vi "2d3dmain.vi"(8 "error in":errorcluster) -> (0 "error out":errorcluster)   [LabVIEW 2023]
uses:
  control/Data Form.ctl
  <vilib>/Utility/miscctls.llb/LVStringsAndValuesArrayTypeDef_U16.ctl
  control/param_calibrazione.ctl
  <vilib>/Analysis/1siggen.llb/Ramp Pattern by Samples.vi
  <vilib>/Utility/file.llb/Read Delimited Spreadsheet (string).vi
  <vilib>/Utility/file.llb/Read Delimited Spreadsheet (DBL).vi
  <vilib>/Utility/file.llb/Write Delimited Spreadsheet (I64).vi
  queue/Front Panel Message Queue.lvlib
  <vilib>/Analysis/NI_AALBase.lvlib
panel:
  in  "Crop Z sl":cluster{i32, i32}(slide) scale=0.0..10.0
  in  "crop Z":bool
  in  "export":bool
  out "deleted portion 2":string
  out "deleted portion":dbl[](array[numeric])
  in  "reset ROI":bool
  in  "save all":bool
  in  "save":bool
  in  "roi":bool
  out "Invert Roi XY":bool[](array[boolean])
  out "Roi XY":T1
  in  "crop all":bool
  in  "crop":bool
  in  "manipulate files":bool
  in  "mapping":enum16{"Y - Linear", "Y - Log"}(ring)
  out "Intensity Graph":i32[][](graph)
  in  "Z Slice":i16(slide) scale=0.0..10.0
  in  "load param":bool
  in  "load calib":bool
  in  "ROIs List":i16(ring) items=["New", "Unknown - Unknown", "Al - Ka1", "Si - Ka1", "Ca - Escape Peak", "S - Ka1", "Cl - Ka1", "Ar - Ka1", "Ar - Kb1", "K - Ka1", "Ca - Ka1", "Ca - Kb1", "Ti - Ka1", "Ti - Kb1", "Cr - Ka1", "Mn - Ka1", "Fe - Ka1", "Fe - Kb1", "Ni - Ka1", "Cu - Ka1", "Zn - Ka1", "Zn - Kb1", "Pb - La1", "Pb - Lb2"]
  in  "calibrate":bool
  out "XY Graph":cluster{"Ramp Pattern":dbl[], i32[]}(graph)
  in  "load data":bool
  in  "Data Form":T2={"Dimensions"={"Dim X"=0, "Dim Y"=0, "Dim Z"=0}, "Folder XRF Files"=path "", "Dynamic Load"=FALSE, "Data From Vitruvio?"=TRUE}
  in  "Stop":bool
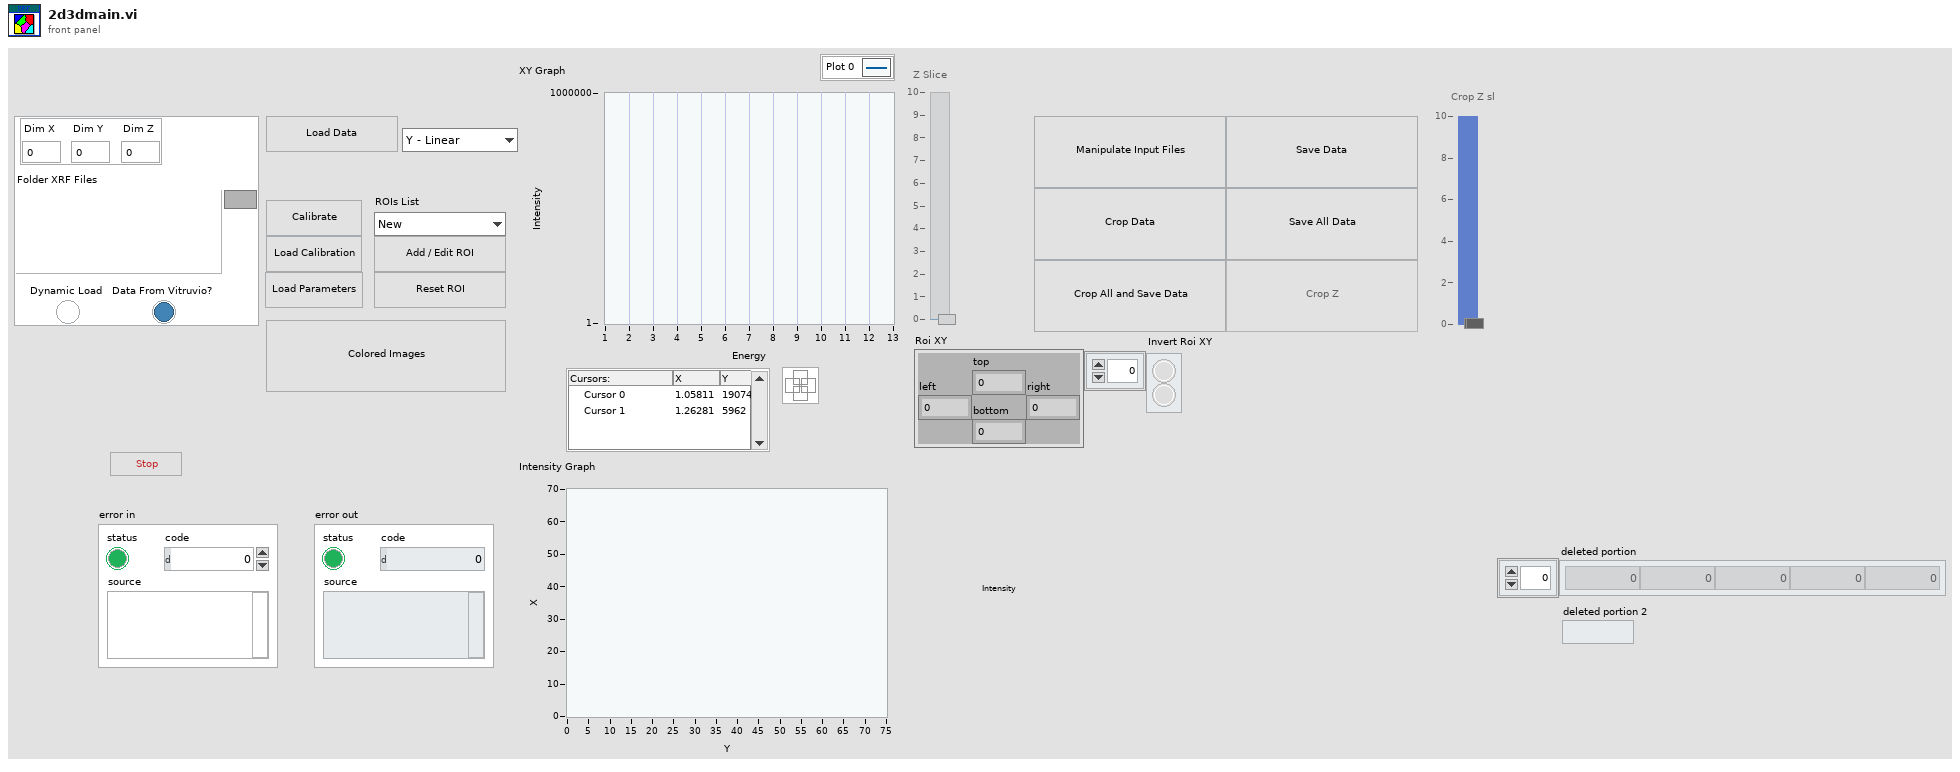
[diagram p1: front panel]
types:
  T1 = cluster{"left":i16, "top":i16, "right":i16, "bottom":i16}
  T2 = typedef "Data Form.ctl" = cluster{"Dimensions":cluster{"Dim X":i32, "Dim Y":i32, "Dim Z":i32}, "Folder XRF Files":path, "Dynamic Load":bool, "Data From Vitruvio?":bool}
  T3 = typedef "Front Panel Message Queue.lvlib/2d3d Message Queues.ctl" = cluster{"Main":refnum<queue>, "2d":refnum<queue>, "3d":refnum<queue>}
  T4 = enum8{"Enabled", "Disabled", "Disabled and Grayed Out"}
  T5 = typedef "param_calibrazione.ctl" = cluster{"Intercept":dbl, "slope":dbl}
  T6 = typedef "LVStringsAndValuesArrayTypeDef_U16.ctl" = cluster{"String":string, "Value":u16}[]
  T7 = typedef "LVCursorListTypeDef.ctl" = cluster{"Name":string, "Color":u32, "Style":u8, "Point Style":u8, "Name Visible":bool, "Allow Drag":bool, "Cursor Mode":u32, "Plot":i32, "Index":i32, "Position":cluster{"X":dbl, "Y":dbl}, "X Scale":u32, "Y Scale":u32, "Watch Plots":i32[], "Watch All Plots":bool, "Plot Area":i32, "Label Offset":cluster{"X":dbl, "Y":dbl}}[]
  T8 = cluster{"Name":string, "Color":u32, "Style":u8, "Point Style":u8, "Name Visible":bool, "Allow Drag":bool, "Cursor Mode":u32, "Plot":i32, "Index":i32, "Position":cluster{"X":dbl, "Y":dbl}, "X Scale":u32, "Y Scale":u32, "Watch Plots":i32[], "Watch All Plots":bool, "Plot Area":i32, "Label Offset":cluster{"X":dbl, "Y":dbl}}
  T9 = cluster{"Name":string, "Color":u32, "Style":u8, "Point Style":u8, "Name Visible":bool, "Allow Drag":bool, "Cursor Mode":u32, "Plot":i32, "Index":i32, "Position":cluster{"X":dbl, "Y":dbl}, "X Scale":u32, "Y Scale":u32, "Watch Plots":i32[], "Watch All Plots":bool, "Plot Area":i32, "Label Offset":cluster{"X":dbl, "Y":dbl}}[]
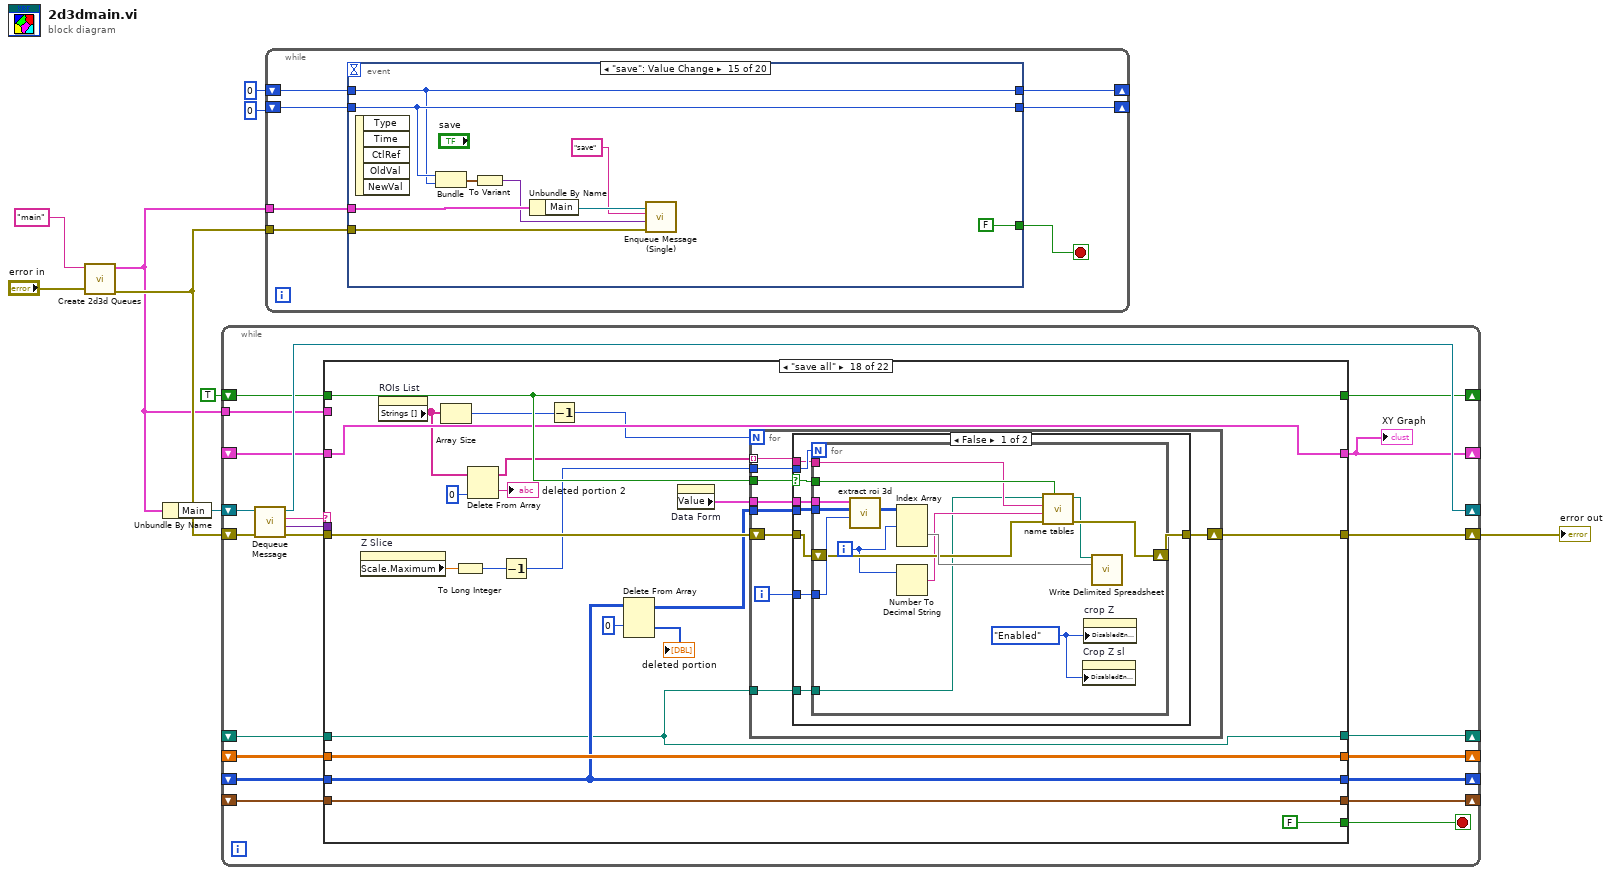
[diagram p0: block diagram]
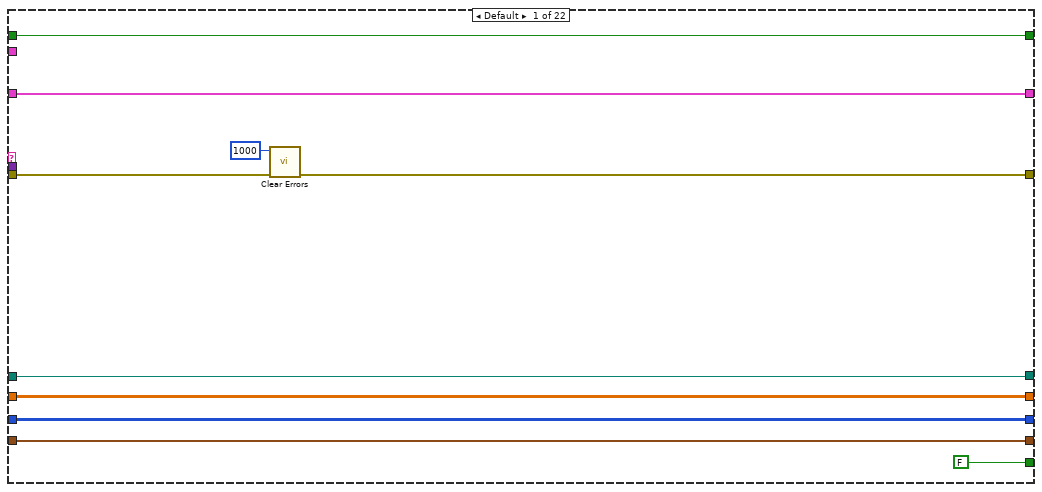
[diagram p2: hidden frame]
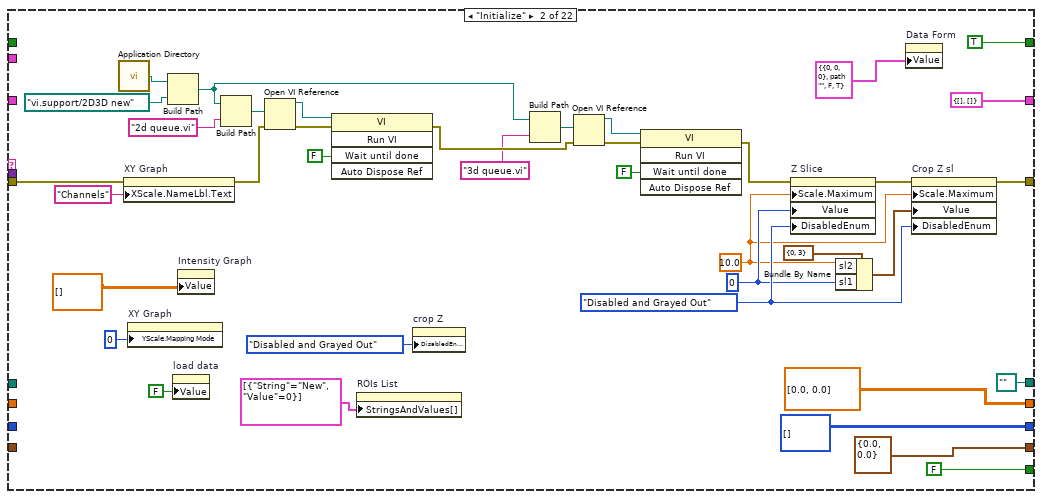
[diagram p3: hidden frame]
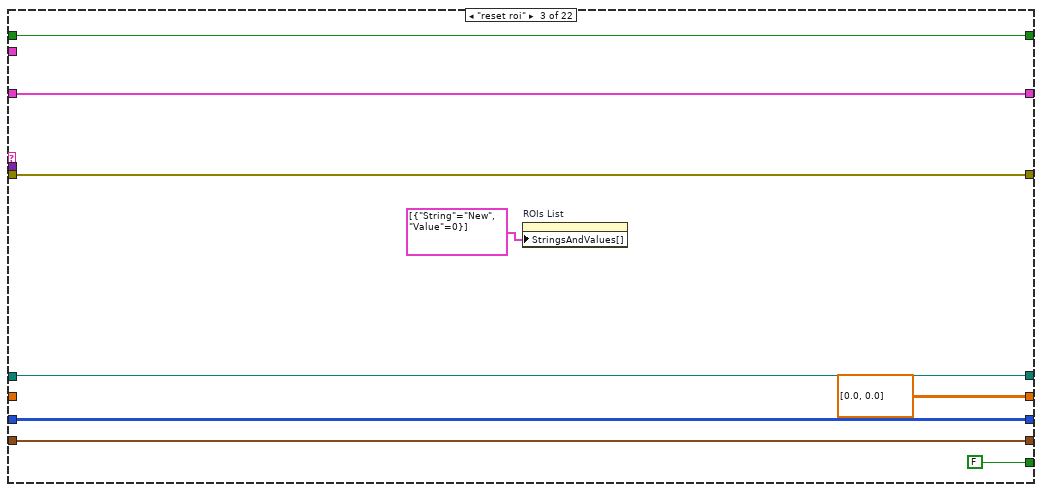
[diagram p4: hidden frame]
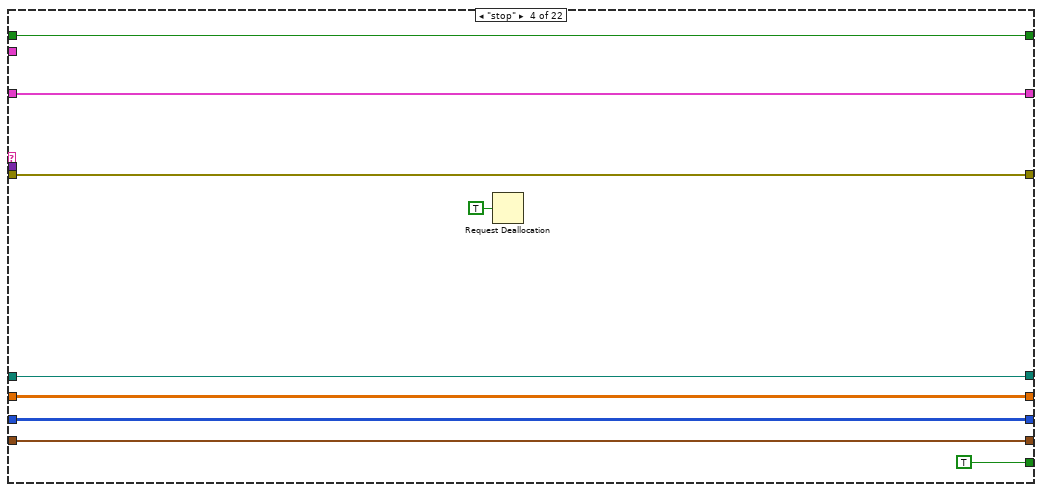
[diagram p5: hidden frame]
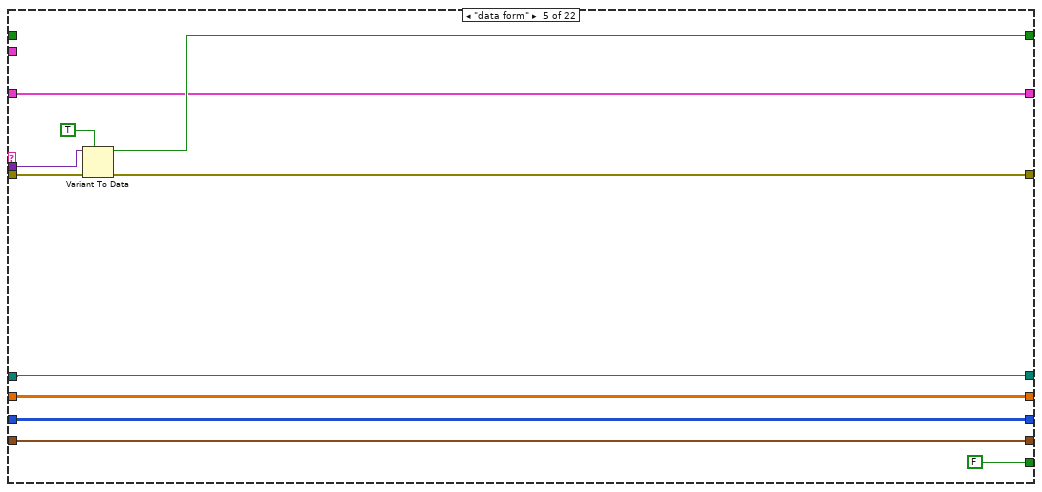
[diagram p6: hidden frame]
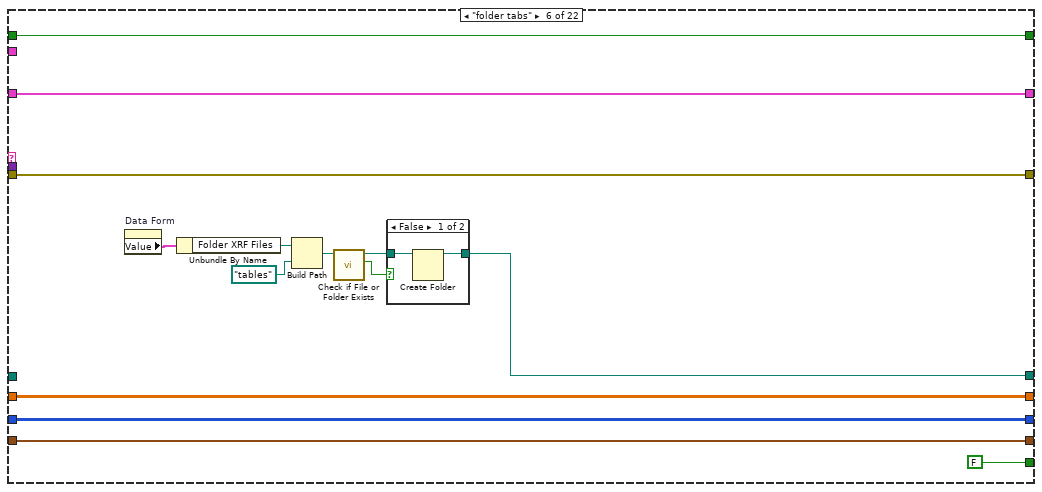
[diagram p7: hidden frame]
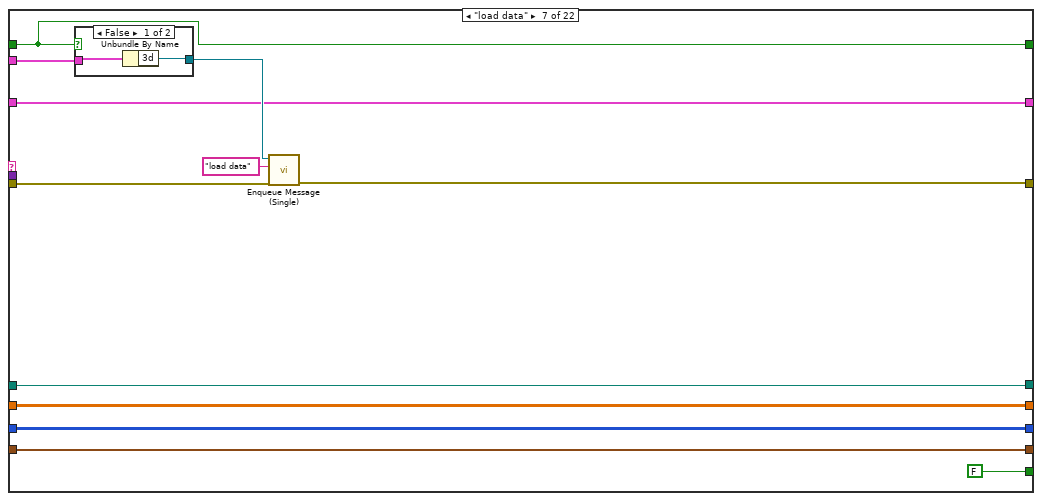
[diagram p9: hidden frame]
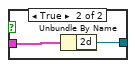
[diagram p10: hidden frame]
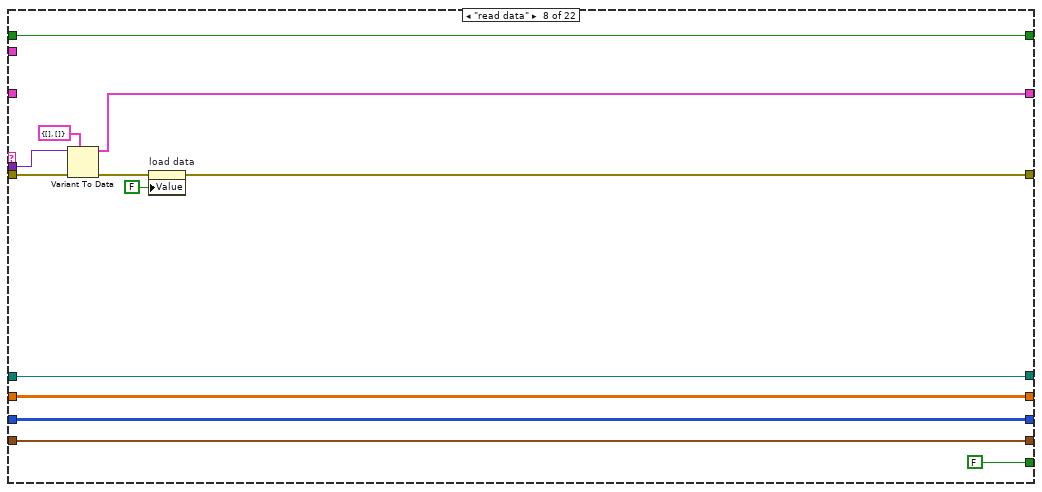
[diagram p11: hidden frame]
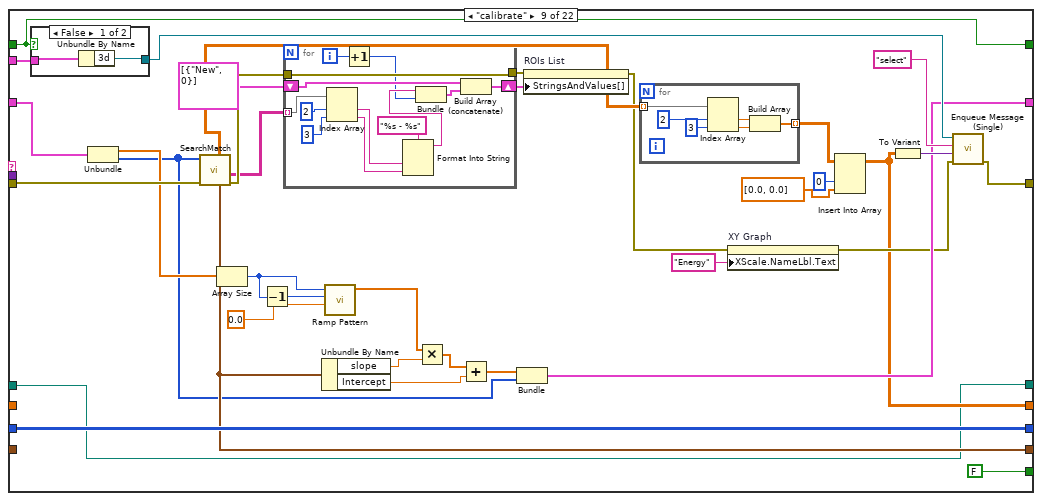
[diagram p12: hidden frame]
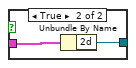
[diagram p13: hidden frame]
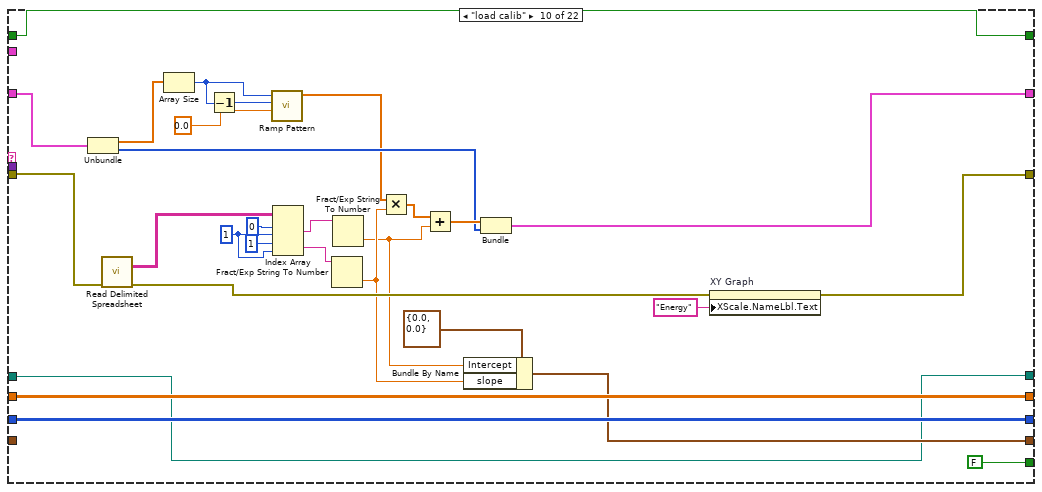
[diagram p14: hidden frame]
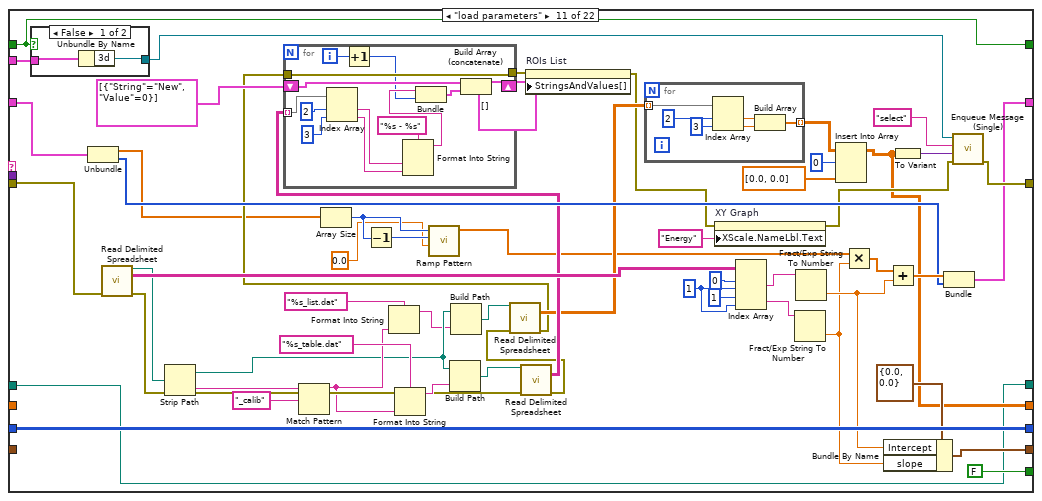
[diagram p15: hidden frame]
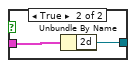
[diagram p16: hidden frame]
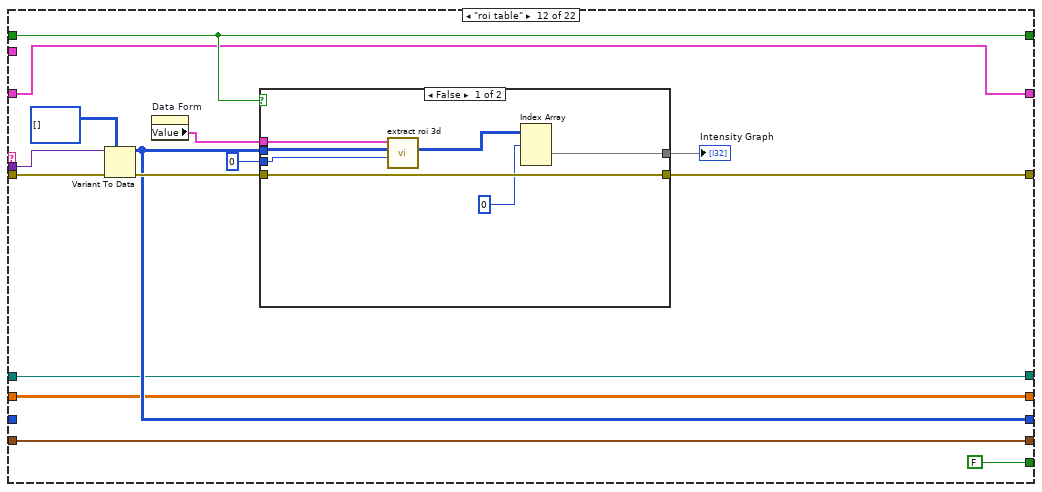
[diagram p17: hidden frame]
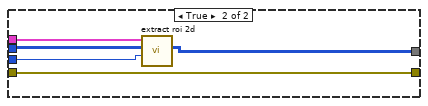
[diagram p18: hidden frame]
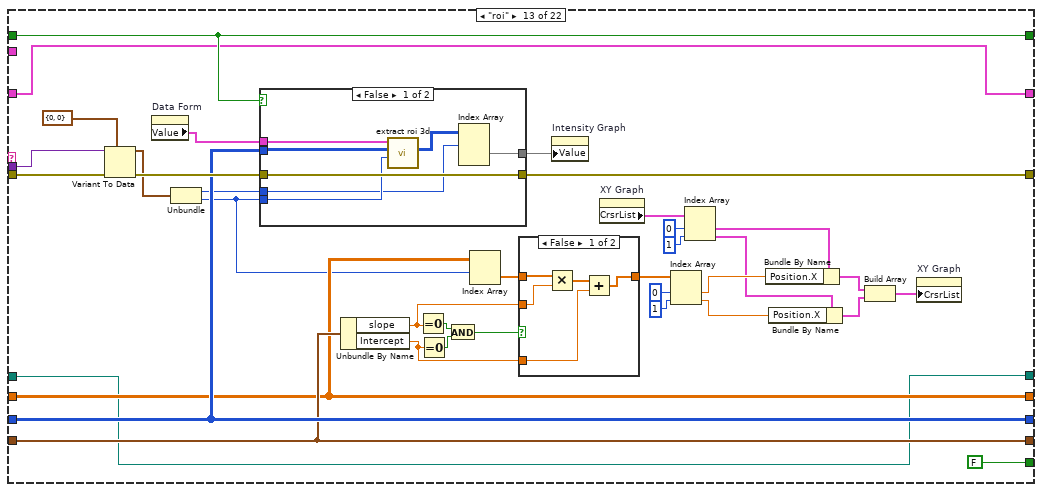
[diagram p19: hidden frame]
diagram:
  n1 = call "Create 2d3d Queues.vi"("error in (no error)"="error in", "name"="main") -> ("error out"=w7:errorcluster, "Message Queues"=w3:T3)  [unwired: 8 in]
  n2 = Unbundle By Name(w3) -> ("Main"=w6:refnum<queue>)
  n3 = while {
    shift-right: [w28] -> _
    shift-left: w6 -> [w29]
    shift-right: [w25] -> w5
    shift-left: w7 -> [w30]
    shift-right: [w21] -> _
    shift-left: TRUE -> [w22]
    tunnel: w3 -> [w20]
    shift-right: [w16] -> _
    shift-left: _ -> [w19]
    shift-right: [w18] -> _
    shift-left: _ -> [w17]
    shift-right: [w15] -> _
    shift-left: _ -> [w14]
    shift-right: [w13] -> _
    shift-left: _ -> [w12]
    shift-right: [w11] -> _
    shift-left: _ -> [w10]
    stop <- w24 stop-if-true
    n4 = call "Dequeue Message.vi"("error in (no error)"=w30, "Message Queue"=w29) -> ("error out"=w26:errorcluster, "Message Data"=w23:variant, "Message"=w27:string, "dup Message Queue"=w28:refnum<queue>)  [unwired: 5 in, 1 out]
    n5 = case shown="\"save all\"" w27 {
      tunnel: w26 -> [w35 w58 w83 w96 w107 w121 w134 w152 w188 w228 w276 w334 w382 w424 w470 w497 w541 w617 w672 w683 w696 w704]
      tunnel: [w34 w48 w83 w96 w103 w121 w131 w144 w175 w224 w287 w327 w376 w428 w457 w492 w537 w613 w663 w681 w695 w703] -> w25
      tunnel: [FALSE FALSE FALSE TRUE FALSE FALSE FALSE FALSE FALSE FALSE FALSE FALSE FALSE FALSE FALSE FALSE FALSE FALSE FALSE FALSE FALSE FALSE] -> w24
      tunnel: w23 -> [_ _ _ _ w106 _ _ w151 _ _ _ w333 w381 w425 w469 _ _ _ w671 w682 _ _]
      tunnel: w22 -> [w39 _ w84 w94 _ w108 w130 w150 w179 w239 w291 w331 w380 w432 w468 w496 w540 w616 w669 w687 w694 w701]
      tunnel: [w39 TRUE w84 w94 w104 w108 w130 w150 w179 w239 w291 w331 w380 w432 w468 w496 w540 w616 w669 w687 w694 w701] -> w21
      tunnel: w20 -> [_ _ _ _ _ _ w135 _ w181 _ w292 _ _ w433 _ _ _ _ _ _ _ _]
      tunnel: [w38 cluster{"Ramp Pattern":dbl[], i32[]} {"Ramp Pattern"=[], []} ("output cluster") w85 w93 w98 w112 w129 w148 w170 w235 w283 w329 w378 w422 w466 w495 w539 w615 w668 w686 w697 w702] -> w16
      tunnel: w19 -> [w38 _ w85 w93 w98 w112 w129 _ w187 w240 w296 w329 w378 w422 w466 w495 w539 w615 w668 w686 w697 w702]
      tunnel: [w37 i32[][] [] w82 w92 w101 w119 w128 w147 w169 w227 w259 w325 w374 w427 w464 w493 w524 w605 w666 w685 w698 w706] -> w18
      tunnel: w17 -> [w37 _ w82 w92 w101 w119 w128 w147 w169 w227 w259 _ w374 w427 w464 w493 w524 w605 w666 w685 w698 w706]
      tunnel: [w36 dbl[][] [[0.0, 0.0]] dbl[][] [[0.0, 0.0]] w91 w100 w118 w127 w143 w157 w223 w245 w323 w353 w413 w454 w486 w530 w608 w667 w676 w693 w705] -> w15
      tunnel: w14 -> [w36 _ _ w91 w100 w118 w127 w143 _ w223 _ w323 w353 w423 w454 w486 w530 w608 w667 w676 w693 w705]
      tunnel: [w32 T5 {"Intercept"=0.0, "slope"=0.0} ("Param Calibrazione") w86 w90 w99 w117 w126 w142 w160 w214 w249 w322 w354 w412 w453 w485 w529 w607 w665 w675 w692 w707] -> w13
      tunnel: w12 -> [w32 _ w86 w90 w99 w117 w126 w142 _ _ _ w322 w354 w412 w453 w485 w529 w607 w665 w675 w692 w707]
      tunnel: [w31 path "" ("dup path") w79 w88 w97 w109 w125 w141 w155 w213 w242 w321 w348 w402 w452 w484 w528 w597 w662 w674 w691 w700] -> w11
      tunnel: w10 -> [w31 _ w79 w88 w97 _ w125 w141 w155 w213 w242 w321 w348 w402 w452 w484 w528 w597 w662 w674 w691 w700]
      frame Default {
        n6 = call <vilib>:"Clear Errors.vi"("error in (no error)"=w35, "specific error code to clear (0: all)"=1000) -> ("error out"=w34:errorcluster)  [unwired: 4 in, 1 out]
      }
      frame "Initialize" {
        w46 = T4."Disabled and Grayed Out" ("Disabled")
        w43 = 0 ("Z Slice")
        w41 = 10.0 ("Scale.Range:Maximum")
        n7 = call <vilib>:"Application Directory.vi"() -> ("Application Directory"=w77:path)
        n8 = property on="XY Graph" class="XYGraph (strict)"(error in=w58, "XScale.NameLbl.Text"="Channels" ("X Scale.Name Label.Text")) -> (error out=w57:errorcluster)  [unwired: 1 in, 1 out]
        n9 = property on="XY Graph" class="XYGraph (strict)"("YScale.Mapping Mode"=u8 0 ("Y Scale.Mapping Mode")) -> ()  [unwired: 2 in, 2 out]
        n10 = Build Path(base path=w77, name or relative path=path "vi.support/2D3D new") -> (appended path=w64:path)
        n11 = property on="load data" class="Bool (strict)"("Value"=FALSE ("load data")) -> ()  [unwired: 2 in, 2 out]
        n12 = property on="Intensity Graph" class="IntGraph (strict)"("Value"=dbl[][] []) -> ()  [unwired: 2 in, 2 out]
        n13 = Build Path(base path=w64, name or relative path="2d queue.vi") -> (appended path=w74:path)
        n14 = Open VI Reference(vi path=w74, error in (no error)=w57) -> (vi reference=w73:refnum<vi>, error out=w72:errorcluster)  [unwired: 4 in]
        n15 = invoke class="VI" method="Run VI"(reference=w73, error in=w72, "Wait until done"=FALSE ("Wait Until Done")) -> (error out=w66:errorcluster)  [unwired: 2 in, 4 out]
        n16 = property on="ROIs List" class="Ring (strict)"("StringsAndValues[]"=T6 [{"String"="New", "Value"=0}] ("Strings And Values []")) -> ()  [unwired: 2 in, 2 out]
        n17 = property on="crop Z" class="Bool"("DisabledEnum"=T4."Disabled and Grayed Out" ("Disabled")) -> ()  [unwired: 2 in, 2 out]
        n18 = Build Path(base path=w64, name or relative path="3d queue.vi") -> (appended path=w67:path)
        n19 = Open VI Reference(vi path=w67, error in (no error)=w66) -> (vi reference=w68:refnum<vi>, error out=w69:errorcluster)  [unwired: 4 in]
        n20 = invoke class="VI" method="Run VI"(reference=w68, error in=w69, "Wait until done"=FALSE ("Wait Until Done")) -> (error out=w60:errorcluster)  [unwired: 2 in, 4 out]
        n21 = property on="Z Slice" class="Slide (strict)"(error in=w60, "Scale.Maximum"=w41, "Value"=w43, "DisabledEnum"=w46) -> (error out=w47:errorcluster)  [unwired: 1 in, 1 out]
        n22 = Bundle By Name(cluster=cluster{"sl1":i32, "sl2":i32} {"sl1"=0, "sl2"=3} ("Crop Z"), "sl2"=w41, "sl1"=w43) -> (w42:cluster{"sl1":i32, "sl2":i32})
        n23 = property on="Data Form" class="Clust (strict)"("Value"=T2 {"Dimensions"={"Dim X"=0, "Dim Y"=0, "Dim Z"=0}, "Folder XRF Files"=path "", "Dynamic Load"=FALSE, "Data From Vitruvio?"=TRUE} ("Data Form")) -> ()  [unwired: 2 in, 2 out]
        n24 = property on="Crop Z sl" class="Slide (strict)"(error in=w47, "Scale.Maximum"=w41, "Value"=w42, "DisabledEnum"=w46) -> (error out=w48:errorcluster)  [unwired: 1 in, 1 out]
      }
      frame "reset roi" {
        n25 = property on="ROIs List" class="Ring (strict)"("StringsAndValues[]"=T6 [{"String"="New", "Value"=0}] ("Strings And Values []")) -> ()  [unwired: 2 in, 2 out]
      }
      frame "stop" {
        n26 = Request Deallocation(TRUE ("flag")) -> ()
      }
      frame "data form" {
        n27 = Variant To Data(error in=w107, type=TRUE, Variant=w106) -> (data=w104:bool, error out=w103:errorcluster)
      }
      frame "folder tabs" {
        n28 = property on="Data Form" class="Clust (strict)"() -> ("Value"=w111:T2)  [unwired: 2 in, 2 out]
        n29 = Unbundle By Name(w111) -> ("Folder XRF Files"=w110:path)
        n30 = Build Path(base path=w110, name or relative path=path "tables") -> (appended path=w116:path)
        n31 = call <vilib>:"Check if File or Folder Exists.vi"("path"=w116) -> ("file or folder exists?"=w114:bool, "dup path"=w115:path)  [unwired: 8 in, 1 out]
        n32 = case shown="False" w114 {
          tunnel: w115 -> [w123 w124]
          tunnel: [w122 w124] -> w109
          frame False {
            n33 = Create Folder(path (use dialog)=w123) -> (created path=w122:path)  [unwired: 2 in, 2 out]
          }
          frame True {
          }
        }
      }
      frame "load data" {
        n34 = case shown="False" w130 {
          tunnel: [w137 w140] -> w133
          tunnel: w135 -> [w138 w139]
          frame False {
            n35 = Unbundle By Name(w138) -> ("3d"=w137:refnum<queue>)
          }
          frame True {
            n36 = Unbundle By Name(w139) -> ("2d"=w140:refnum<queue>)
          }
        }
        n37 = call "Enqueue Message (Single).vi"("error in (no error)"=w134, "Message"="load data", "Message Queue"=w133) -> ("error out"=w131:errorcluster)  [unwired: 7 in, 1 out]
      }
      frame "read data" {
        n38 = Variant To Data(error in=w152, type=cluster{"Ramp Pattern":dbl[], i32[]} {"Ramp Pattern"=[], []} ("output cluster"), Variant=w151) -> (data=w148:cluster{"Ramp Pattern":dbl[], i32[]}, error out=w145:errorcluster)
        n39 = property on="load data" class="Bool (strict)"(error in=w145, "Value"=FALSE ("load data")) -> (error out=w144:errorcluster)  [unwired: 1 in, 1 out]
      }
      frame "calibrate" {
        n40 = case shown="False" w179 {
          tunnel: [w196 w199] -> w178
          tunnel: w181 -> [w197 w198]
          frame False {
            n41 = Unbundle By Name(w197) -> ("3d"=w196:refnum<queue>)
          }
          frame True {
            n42 = Unbundle By Name(w198) -> ("2d"=w199:refnum<queue>)
          }
        }
        n43 = Unbundle(w187) -> ("Ramp Pattern"=w162:dbl[], w154:i32[])
        n44 = call "SearchMatch.vi"("Error In"=w188, "data_from2d3d"=w154) -> ("Error Out"=w186:errorcluster, "Elements Selected"=w184:string[][], "Param Calibrazione"=w160:T5, "List ROI out"=w180:dbl[][])  [unwired: 5 in, 1 out]
        n45 = Array Size(array=w162) -> (size(s)=w165:i32)
        n46 = Decrement(x=w165) -> (x-1=w164:i32)
        n47 = for {
          tunnel: w184 -> [w208] mode=indexing
          shift-right: [w211] -> w182
          shift-left: T6 [{"String"="New", "Value"=0}] ("Strings And Values []") -> [w210]
          tunnel: w186 -> [w206]
          tunnel: [w206] -> w183
          i -> [w209]
          n48 = Index Array(array=w208, index #1=2 ("index"), index #2=3 ("index")) -> (element #1=w203:string, element #2=w202:string)
          n49 = Increment(x=w209) -> (x+1=w200:i32)
          n50 = Format Into String(format string="%s - %s", w203, w202) -> (resulting string=w201:string)  [unwired: 2 in, 1 out]
          n51 = Bundle(w201, w200) -> (w212:cluster{string, i32})  [unwired: 1 in]
          n52 = Build Array (concatenate)(w210, w212) -> (w211:cluster{"String":string, "Value":i32}[])
        }
        n53 = Unbundle By Name(w160) -> ("slope"=w174:dbl, "Intercept"=w172:dbl)
        n54 = call-poly <vilib>:"Ramp Pattern.vi"("start"=0.0, "end"=w164, "samples"=w165) -> ("Ramp Pattern"=w161:dbl[])  [unwired: 7 in, 1 out]
        n55 = Multiply(x=w161, y=w174) -> (x*y=w173:dbl[])
        n56 = Add(x=w173, y=w172) -> (x+y=w171:dbl[])
        n57 = Bundle(w171, w154) -> (w170:cluster{dbl[], i32[]})  [unwired: 1 in]
        n58 = property on="ROIs List" class="Ring (strict)"(error in=w183, "StringsAndValues[]"=w182) -> (error out=w167:errorcluster)  [unwired: 1 in, 1 out]
        n59 = for {
          tunnel: w180 -> [w195] mode=indexing
          tunnel: [w190] -> w156 mode=indexing
          n60 = Index Array(array=w195, index #1=2 ("index"), index #2=3 ("index")) -> (element #1=w191:dbl, element #2=w192:dbl)
          n61 = Build Array(w191, w192) -> (w190:dbl[])
        }
        n62 = property on="XY Graph" class="XYGraph (strict)"(error in=w167, "XScale.NameLbl.Text"="Energy" ("X Scale.Name Label.Text")) -> (error out=w166:errorcluster)  [unwired: 1 in, 1 out]
        n63 = Insert Into Array(array=w156, index (col)=0 ("disabled index (col)"), new element=dbl[] [0.0, 0.0]) -> (w157:dbl[][])  [unwired: 1 in]
        n64 = To Variant(anything=w157) -> (Variant=w177:variant)
        n65 = call "Enqueue Message (Single).vi"("error in (no error)"=w166, "Message Data"=w177, "Message"="select", "Message Queue"=w178) -> ("error out"=w175:errorcluster)  [unwired: 6 in, 1 out]
      }
      frame "load calib" {
        w232 = 1 ("disabled index (col)")
        n66 = Unbundle(w240) -> ("Ramp Pattern"=w219:dbl[], w236:i32[])
        n67 = call-poly <vilib>:"Read Delimited Spreadsheet.vi"("error in (no error)"=w228) -> ("all rows"=w229:string[][], "error out"=w225:errorcluster)  [unwired: 9 in, 4 out]
        n68 = Array Size(array=w219) -> (size(s)=w222:i32)
        n69 = Decrement(x=w222) -> (x-1=w221:i32)
        n70 = call-poly <vilib>:"Ramp Pattern.vi"("start"=0.0, "end"=w221, "samples"=w222) -> ("Ramp Pattern"=w218:dbl[])  [unwired: 7 in, 1 out]
        n71 = Index Array(array=w229, index (row) #1=0 ("index (row)"), index (col) #1=w232, index (row) #2=1 ("index (row)"), index (col) #2=w232) -> (element #1=w233:string, element #2=w234:string)
        n72 = Fract/Exp String To Number(string=w234) -> (number=w216:dbl)  [unwired: 3 in, 1 out]
        n73 = Fract/Exp String To Number(string=w233) -> (number=w215:dbl)  [unwired: 3 in, 1 out]
        n74 = Multiply(x=w218, y=w216) -> (x*y=w238:dbl[])
        n75 = Add(x=w238, y=w215) -> (x+y=w237:dbl[])
        n76 = Bundle By Name(cluster=T5 {"Intercept"=0.0, "slope"=0.0} ("Param Calibrazione"), "Intercept"=w215, "slope"=w216) -> (w214:T5)
        n77 = Bundle(w237, w236) -> (w235:cluster{dbl[], i32[]})  [unwired: 1 in]
        n78 = property on="XY Graph" class="XYGraph (strict)"(error in=w225, "XScale.NameLbl.Text"="Energy" ("X Scale.Name Label.Text")) -> (error out=w224:errorcluster)  [unwired: 1 in, 1 out]
      }
      frame "load parameters" {
        (unwired) cluster{"String":string, "Value":i32}[] [] ("Strings And Values []")
        w280 = 1 ("disabled index (col)")
        n79 = case shown="False" w291 {
          tunnel: [w304 w307] -> w290
          tunnel: w292 -> [w305 w306]
          frame False {
            n80 = Unbundle By Name(w305) -> ("3d"=w304:refnum<queue>)
          }
          frame True {
            n81 = Unbundle By Name(w306) -> ("2d"=w307:refnum<queue>)
          }
        }
        n82 = Unbundle(w296) -> ("Ramp Pattern"=w252:dbl[], w284:i32[])
        n83 = call-poly <vilib>:"Read Delimited Spreadsheet.vi"("error in (no error)"=w276) -> ("new file path (Not A Path if cancelled)"=w274:path, "all rows"=w277:string[][], "error out"=w269:errorcluster)  [unwired: 9 in, 3 out]
        n84 = Strip Path(path=w274) -> (stripped path=w265:path, name=w268:string)
        n85 = Match Pattern(string=w268, regular expression="_calib" ("format string")) -> (before substring=w266:string)  [unwired: 1 in, 3 out]
        n86 = Array Size(array=w252) -> (size(s)=w255:i32)
        n87 = Decrement(x=w255) -> (x-1=w254:i32)
        n88 = Format Into String(format string="%s_list.dat", w266) -> (resulting string=w264:string)  [unwired: 2 in, 1 out]
        n89 = Format Into String(format string="%s_table.dat", w266) -> (resulting string=w272:string)  [unwired: 2 in, 1 out]
        n90 = call-poly <vilib>:"Ramp Pattern.vi"("start"=0.0, "end"=w254, "samples"=w255) -> ("Ramp Pattern"=w251:dbl[])  [unwired: 7 in, 1 out]
        n91 = Build Path(base path=w265, name or relative path=w272) -> (appended path=w271:path)
        n92 = Build Path(base path=w265, name or relative path=w264) -> (appended path=w263:path)
        n93 = call-poly <vilib>:"Read Delimited Spreadsheet.vi"("file path (dialog if empty)"=w271, "error in (no error)"=w269) -> ("all rows"=w270:string[][], "error out"=w261:errorcluster)  [unwired: 8 in, 4 out]
        n94 = call-poly <vilib>:"Read Delimited Spreadsheet.vi"("file path (dialog if empty)"=w263, "error in (no error)"=w261) -> ("all rows"=w262:dbl[][], "error out"=w260:errorcluster)  [unwired: 8 in, 4 out]
        n95 = for {
          tunnel: w270 -> [w316] mode=indexing
          shift-right: [w319] -> w293
          shift-left: T6 [{"String"="New", "Value"=0}] ("Strings And Values []") -> [w318]
          tunnel: w260 -> [w314]
          tunnel: [w314] -> w294
          i -> [w317]
          n96 = Index Array(array=w316, index #1=2 ("index"), index #2=3 ("index")) -> (element #1=w311:string, element #2=w310:string)
          n97 = Increment(x=w317) -> (x+1=w308:i32)
          n98 = Format Into String(format string="%s - %s", w311, w310) -> (resulting string=w309:string)  [unwired: 2 in, 1 out]
          n99 = Bundle(w309, w308) -> (w320:cluster{string, i32})  [unwired: 1 in]
          n100 = Build Array (concatenate)(w318, w320) -> (w319:cluster{"String":string, "Value":i32}[])
        }
        n101 = property on="ROIs List" class="Ring (strict)"(error in=w294, "StringsAndValues[]"=w293) -> (error out=w257:errorcluster)  [unwired: 1 in, 1 out]
        n102 = for {
          tunnel: w262 -> [w303] mode=indexing
          tunnel: [w298] -> w244 mode=indexing
          n103 = Index Array(array=w303, index #1=2 ("index"), index #2=3 ("index")) -> (element #1=w299:dbl, element #2=w300:dbl)
          n104 = Build Array(w299, w300) -> (w298:dbl[])
        }
        n105 = property on="XY Graph" class="XYGraph (strict)"(error in=w257, "XScale.NameLbl.Text"="Energy" ("X Scale.Name Label.Text")) -> (error out=w256:errorcluster)  [unwired: 1 in, 1 out]
        n106 = Index Array(array=w277, index (row) #1=0 ("index (row)"), index (col) #1=w280, index (row) #2=1 ("index (row)"), index (col) #2=w280) -> (element #1=w281:string, element #2=w282:string)
        n107 = Fract/Exp String To Number(string=w282) -> (number=w247:dbl)  [unwired: 3 in, 1 out]
        n108 = Fract/Exp String To Number(string=w281) -> (number=w248:dbl)  [unwired: 3 in, 1 out]
        n109 = Insert Into Array(array=w244, index (row)=0 ("disabled index (col)"), new element=dbl[] [0.0, 0.0]) -> (w245:dbl[][])  [unwired: 1 in]
        n110 = Multiply(x=w251, y=w247) -> (x*y=w286:dbl[])
        n111 = Bundle By Name(cluster=T5 {"Intercept"=0.0, "slope"=0.0} ("Param Calibrazione"), "Intercept"=w248, "slope"=w247) -> (w249:T5)
        n112 = Add(x=w286, y=w248) -> (x+y=w285:dbl[])
        n113 = To Variant(anything=w245) -> (Variant=w289:variant)
        n114 = Bundle(w285, w284) -> (w283:cluster{dbl[], i32[]})  [unwired: 1 in]
        n115 = call "Enqueue Message (Single).vi"("error in (no error)"=w256, "Message Data"=w289, "Message"="select", "Message Queue"=w290) -> ("error out"=w287:errorcluster)  [unwired: 6 in, 1 out]
      }
      frame "roi table" {
        n116 = Variant To Data(error in=w334, type=i32[][] [], Variant=w333) -> (data=w325:i32[][], error out=w330:errorcluster)
        n117 = property on="Data Form" class="Clust (strict)"() -> ("Value"=w328:T2)  [unwired: 2 in, 2 out]
        n118 = case shown="False" w331 {
          tunnel: w325 -> [w342 w346]
          tunnel: w330 -> [w340 w345]
          tunnel: w328 -> [w341 w347]
          tunnel: [w340 w345] -> w327
          tunnel: [w338 w344] -> w326
          tunnel: i16 0 ("ROI selected") -> [w337 w343]
          frame False {
            n119 = call "extract roi 3d.vi"("ROI selected"=w337, "ROIs Array In"=w342, "Data Form"=w341) -> ("Table ROI 3D"=w339:i32[][][])  [unwired: 8 in]
            n120 = Index Array(array=w339, index (dim 0)=i16 0) -> (element=w338:i32[][])  [unwired: 2 in]
          }
          frame True {
            n121 = call "extract roi 2d.vi"("ROI selected"=w343, "ROIs Array In"=w346, "Data Form"=w347) -> ("Table ROI 2D"=w344:i32[][])  [unwired: 8 in]
          }
        }
        "Intensity Graph" <- w326
      }
      frame "roi" {
        n122 = Variant To Data(error in=w382, type=cluster{"NewVal":i16, "ROIs List":i16} {"NewVal"=0, "ROIs List"=0} ("output cluster"), Variant=w381) -> (data=w372:cluster{"NewVal":i16, "ROIs List":i16}, error out=w379:errorcluster)
        n123 = property on="Data Form" class="Clust (strict)"() -> ("Value"=w377:T2)  [unwired: 2 in, 2 out]
        n124 = Unbundle(w372) -> ("NewVal"=w371:i16, "ROIs List"=w349:i16)
        n125 = case shown="False" w380 {
          tunnel: w374 -> [w396 w400]
          tunnel: w379 -> [w394 w399]
          tunnel: w377 -> [w395 w401]
          tunnel: [w394 w399] -> w376
          tunnel: [w392 w398] -> w375
          tunnel: w371 -> [w390 _]
          tunnel: w349 -> [w391 w397]
          frame False {
            n126 = call "extract roi 3d.vi"("ROI selected"=w391, "ROIs Array In"=w396, "Data Form"=w395) -> ("Table ROI 3D"=w393:i32[][][])  [unwired: 8 in]
            n127 = Index Array(array=w393, index (dim 0)=w390) -> (element=w392:i32[][])  [unwired: 2 in]
          }
          frame True {
            n128 = call "extract roi 2d.vi"("ROI selected"=w397, "ROIs Array In"=w400, "Data Form"=w401) -> ("Table ROI 2D"=w398:i32[][])  [unwired: 8 in]
          }
        }
        n129 = Unbundle By Name(w354) -> ("slope"=w365:dbl, "Intercept"=w366:dbl)
        n130 = Equal To 0?(x=w365) -> (x = 0?=w362:bool)
        n131 = Equal To 0?(x=w366) -> (x = 0?=w363:bool)
        n132 = And(x=w362, y=w363) -> (x .and. y?=w364:bool)
        n133 = Index Array(array=w353, index (row)=w349) -> (element=w368:dbl[])  [unwired: 1 in]
        n134 = case shown="False" w364 {
          tunnel: w368 -> [w388 w389]
          tunnel: [w384 w389] -> w367
          tunnel: w365 -> [w387 _]
          tunnel: w366 -> [w385 _]
          frame False {
            n135 = Multiply(x=w388, y=w387) -> (x*y=w386:dbl[])
            n136 = Add(x=w386, y=w385) -> (x+y=w384:dbl[])
          }
          frame True {
          }
        }
        n137 = property on="Intensity Graph" class="IntGraph (strict)"("Value"=w375) -> ()  [unwired: 2 in, 2 out]
        n138 = property on="XY Graph" class="XYGraph (strict)"() -> ("CrsrList"=w359:T7)  [unwired: 2 in, 2 out]
        n139 = Index Array(array=w367, index #1=0 ("index"), index #2=1 ("index")) -> (element #1=w369:dbl, element #2=w370:dbl)
        n140 = Index Array(array=w359, index #1=0 ("index"), index #2=1 ("index")) -> (element #1=w360:T8, element #2=w361:T8)
        n141 = Bundle By Name(cluster=w360, "Position.X"=w369) -> (w352:T8)
        n142 = Bundle By Name(cluster=w361, "Position.X"=w370) -> (w351:T8)
        n143 = Build Array(w352, w351) -> (w350:T9)
        n144 = property on="XY Graph" class="XYGraph (strict)"("CrsrList"=w350) -> ()  [unwired: 2 in, 2 out]
      }
      frame "edit roi" {
        n145 = case shown="True" w432 {
          tunnel: [w448 w451] -> w431
          tunnel: w433 -> [w449 w450]
          frame False {
            n146 = Unbundle By Name(w449) -> ("3d"=w448:refnum<queue>)
          }
          frame True {
            n147 = Unbundle By Name(w450) -> ("2d"=w451:refnum<queue>)
          }
        }
        n148 = property on="XY Graph" class="XYGraph (strict)"() -> ("CrsrList"=w420:T7)  [unwired: 2 in, 2 out]
        n149 = Index Array(array=w420, index #1=0 ("index"), index #2=1 ("index")) -> (element #1=w417:T8, element #2=w404:T8)
        n150 = Variant To Data(error in=w424, type=cluster{"NewVal":i16, "ROIs List":i16, bool} {"NewVal"=0, "ROIs List"=0, FALSE} ("output cluster"), Variant=w425) -> (data=w421:cluster{"NewVal":i16, "ROIs List":i16, bool})  [unwired: 1 out]
        n151 = Unbundle(w421) -> ("ROIs List"=w414:i16, w403:bool)  [unwired: 1 out]
        n152 = Unbundle By Name(w417) -> ("Position.X"=w416:dbl)
        n153 = Unbundle By Name(w404) -> ("Position.X"=w415:dbl)
        n154 = Unbundle By Name(w412) -> ("Intercept"=w406:dbl, "slope"=w405:dbl)
        n155 = Equal To 0?(x=w406) -> (x = 0?=w411:bool)
        n156 = Equal To 0?(x=w405) -> (x = 0?=w410:bool)
        n157 = Build Array(w416, w415) -> (w408:dbl[])
        n158 = And(x=w411, y=w410) -> (x .and. y?=w409:bool)
        n159 = case shown="False" w409 {
          tunnel: w408 -> [w439 w440]
          tunnel: [w435 w440] -> w407
          tunnel: w406 -> [w438 _]
          tunnel: w405 -> [w436 _]
          frame False {
            n160 = Subtract(x=w439, y=w438) -> (x-y=w437:dbl[])
            n161 = Divide(x=w437, y=w436) -> (x/y=w435:dbl[])
          }
          frame True {
          }
        }
        n162 = case shown="False" w403 {
          tunnel: [w444 w447] -> w413
          tunnel: w423 -> [w443 w445]
          tunnel: w407 -> [w442 w446]
          tunnel: w414 -> [w441 _]
          frame False {
            n163 = Replace Array Subset(array=w443, new element=w442, index (row)=w441) -> (w444:dbl[][])  [unwired: 1 in]
          }
          frame True {
            n164 = Build Array (concatenate)(w445, w446) -> (w447:dbl[][])
          }
        }
        n165 = To Variant(anything=w413) -> (Variant=w430:variant)
        n166 = call "Enqueue Message (Single).vi"("Message Data"=w430, "Message"="select", "Message Queue"=w431) -> ("error out"=w428:errorcluster)  [unwired: 7 in, 1 out]
      }
      frame "crop" {
        n167 = Variant To Data(error in=w470, type=cluster{"NewVal":i16, "ROIs List":i16} {"NewVal"=0, "ROIs List"=0} ("output cluster"), Variant=w469) -> (data=w462:cluster{"NewVal":i16, "ROIs List":i16}, error out=w467:errorcluster)
        n168 = property on="Data Form" class="Clust (strict)"() -> ("Value"=w465:T2)  [unwired: 2 in, 2 out]
        n169 = Unbundle(w462) -> ("NewVal"=w459:i16, "ROIs List"=w458:i16)
        n170 = case shown="False" w468 {
          tunnel: w464 -> [w478 w482]
          tunnel: w467 -> [w476 w481]
          tunnel: w465 -> [w477 w483]
          tunnel: [w476 w481] -> w461
          tunnel: [w474 w480] -> w460
          tunnel: w459 -> [w472 _]
          tunnel: w458 -> [w473 w479]
          frame False {
            n171 = call "extract roi 3d.vi"("ROI selected"=w473, "ROIs Array In"=w478, "Data Form"=w477) -> ("Table ROI 3D"=w475:i32[][][])  [unwired: 8 in]
            n172 = Index Array(array=w475, index (dim 0)=w472) -> (element=w474:i32[][])  [unwired: 2 in]
          }
          frame True {
            n173 = call "extract roi 2d.vi"("ROI selected"=w479, "ROIs Array In"=w482, "Data Form"=w483) -> ("Table ROI 2D"=w480:i32[][])  [unwired: 8 in]
          }
        }
        n174 = property on="Intensity Graph" class="IntGraph (strict)"("Value"=w460) -> ()  [unwired: 2 in, 2 out]
        n175 = call "Crop Graph.vi"("error in"=w461, "Image In"=w460) -> ("error out"=w457:errorcluster, "Invert Roi"=→"Invert Roi XY":bool[], "Roi"=→"Roi XY":T1)  [unwired: 7 in]
      }
      frame "save" {
        n176 = property on="Z Slice" class="Slide (strict)"() -> ("Scale.Maximum"=w491:dbl)  [unwired: 2 in, 2 out]
        n177 = property on="ROIs List" class="Ring (strict)"() -> ("Strings []"=w490:string[], "Value"=w488:i16)  [unwired: 2 in, 2 out]
        n178 = Index Array(array=w490, index=w488) -> (element=w489:string)
        n179 = To Long Integer(number=w491) -> (32bit integer=w487:i32)
        n180 = property on="Data Form" class="Clust (strict)"() -> ("Value"=w494:T2)  [unwired: 2 in, 2 out]
        n181 = case shown="False" w496 {
          selector: w496 -> [w508 w517]
          tunnel: w493 -> [w511 w521]
          tunnel: w497 -> [w506 w514]
          tunnel: w494 -> [w510 w516]
          tunnel: [w505 w513] -> w492
          tunnel: w488 -> [w509 w520]
          tunnel: w489 -> [w507 w515]
          tunnel: w487 -> [w504 _]
          tunnel: w484 -> [w499 w512]
          frame False {
            n182 = call "extract roi 3d.vi"("ROI selected"=w509, "ROIs Array In"=w511, "Data Form"=w510) -> ("Table ROI 3D"=w503:i32[][][])  [unwired: 8 in]
            n183 = Index Array(array=w503, index (dim 0)=w504) -> (element=w502:i32[][])  [unwired: 2 in]
            n184 = Number To Decimal String(number=w504) -> (decimal integer string=w501:string)  [unwired: 1 in]
            n185 = call "name tables.vi"("2D?"=w508, "error in"=w506, "Z Slice"=w501, "ROI"=w507, "path folder in"=w499) -> ("error out"=w505:errorcluster, "path file out"=w500:path)  [unwired: 5 in]
            n186 = call-poly <vilib>:"Write Delimited Spreadsheet.vi"("file path (dialog if empty)"=w500, "2D data"=w502) -> ()  [unwired: 12 in, 2 out]
          }
          frame True {
            n187 = call "extract roi 2d.vi"("ROI selected"=w520, "ROIs Array In"=w521, "Data Form"=w516) -> ("Table ROI 2D"=w519:i32[][])  [unwired: 8 in]
            n188 = call "name tables.vi"("2D?"=w517, "error in"=w514, "ROI"=w515, "path folder in"=w512) -> ("error out"=w513:errorcluster, "path file out"=w518:path)  [unwired: 6 in]
            n189 = call-poly <vilib>:"Write Delimited Spreadsheet.vi"("file path (dialog if empty)"=w518, "2D data"=w519) -> ()  [unwired: 12 in, 2 out]
          }
        }
      }
      frame "crop all" {
        n190 = property on="Z Slice" class="Slide (strict)"() -> ("Scale.Maximum"=w536:dbl)  [unwired: 2 in, 2 out]
        n191 = property on="Invert Roi XY" class="Arr (strict)"() -> ("Value"=w532:bool[])  [unwired: 2 in, 2 out]
        n192 = property on="Roi XY" class="Clust (strict)"() -> ("Value"=w531:T1)  [unwired: 2 in, 2 out]
        n193 = property on="ROIs List" class="Ring (strict)"() -> ("Strings []"=w527:string[])  [unwired: 2 in, 2 out]
        n194 = Array Size(array=w527) -> (size(s)=w533:i32)
        n195 = To Long Integer(number=w536) -> (32bit integer=w535:i32)
        n196 = Delete From Array(array=w527, index=0 ("index (row)")) -> (array with subset deleted=w526:string[])  [unwired: 1 in, 1 out]
        n197 = Decrement(x=w535) -> (x-1=w534:i32)
        n198 = property on="Data Form" class="Clust (strict)"() -> ("Value"=w538:T2)  [unwired: 2 in, 2 out]
        n199 = Delete From Array(array=w524, index (row)=0) -> (array with subset deleted=w523:i32[][])  [unwired: 2 in, 1 out]
        n200 = for {
          N: w533 -> [_]
          tunnel: w540 -> [w552]
          tunnel: w538 -> [w551]
          tunnel: w523 -> [w550]
          tunnel: w534 -> [w548]
          shift-right: [w549] -> w537
          shift-left: w541 -> [w553]
          tunnel: w532 -> [w546]
          tunnel: w531 -> [w545]
          tunnel: w526 -> [w544] mode=indexing
          tunnel: w528 -> [w543]
          i -> [w547]
          n201 = case shown="True" w552 {
            selector: w552 -> [w558 w588]
            tunnel: w550 -> [w564 w596]
            tunnel: w553 -> [w556 w585]
            tunnel: w551 -> [w563 w587]
            tunnel: [w555 w584] -> w549
            tunnel: w548 -> [w562 _]
            tunnel: w547 -> [w561 w595]
            tunnel: w546 -> [w559 w591]
            tunnel: w545 -> [w560 w593]
            tunnel: w544 -> [w557 w586]
            tunnel: w543 -> [w554 w583]
            frame False {
              n202 = for {
                N: w562 -> [_]
                tunnel: w564 -> [w582]
                tunnel: w563 -> [w574]
                tunnel: w561 -> [w580]
                tunnel: w560 -> [w576]
                tunnel: w559 -> [w575]
                tunnel: w558 -> [w573]
                tunnel: w557 -> [w572]
                shift-right: [w570] -> w555
                shift-left: w556 -> [w571]
                tunnel: w554 -> [w566]
                i -> [w569]
                w565 = T4."Enabled" ("Disabled")
                n203 = call "extract roi 3d.vi"("ROI selected"=w580, "ROIs Array In"=w582, "Data Form"=w574) -> ("Table ROI 3D"=w581:i32[][][])  [unwired: 8 in]
                n204 = Index Array(array=w581, index (dim 0)=w569) -> (element=w577:i32[][])  [unwired: 2 in]
                n205 = Number To Decimal String(number=w569) -> (decimal integer string=w568:string)  [unwired: 1 in]
                n206 = call "Crop Roi.vi"("Roi"=w576, "Table Roi In"=w577) -> ("Table Roi Out"=w579:i32[][])  [unwired: 9 in]
                n207 = call "Programmatically Invert Roi.vi"("Invert Roi"=w575, "Table Roi In"=w579) -> ("Table Roi Out"=w578:i32[][])  [unwired: 9 in]
                n208 = call "name tables.vi"("2D?"=w573, "error in"=w571, "Z Slice"=w568, "ROI"=w572, "path folder in"=w566) -> ("error out"=w570:errorcluster, "path file out"=w567:path)  [unwired: 5 in]
                n209 = property on="Crop Z sl" class="Slide (strict)"("DisabledEnum"=w565) -> ()  [unwired: 2 in, 2 out]
                n210 = property on="crop Z" class="Bool"("DisabledEnum"=w565) -> ()  [unwired: 2 in, 2 out]
                n211 = call-poly <vilib>:"Write Delimited Spreadsheet.vi"("file path (dialog if empty)"=w567, "2D data"=w578) -> ()  [unwired: 12 in, 2 out]
              }
            }
            frame True {
              n212 = call "extract roi 2d.vi"("ROI selected"=w595, "ROIs Array In"=w596, "Data Form"=w587) -> ("Table ROI 2D"=w594:i32[][])  [unwired: 8 in]
              n213 = call "Crop Roi.vi"("Roi"=w593, "Table Roi In"=w594) -> ("Table Roi Out"=w592:i32[][])  [unwired: 9 in]
              n214 = call "Programmatically Invert Roi.vi"("Invert Roi"=w591, "Table Roi In"=w592) -> ("Table Roi Out"=w590:i32[][])  [unwired: 9 in]
              n215 = call "name tables.vi"("2D?"=w588, "error in"=w585, "ROI"=w586, "path folder in"=w583) -> ("error out"=w584:errorcluster, "path file out"=w589:path)  [unwired: 6 in]
              n216 = call-poly <vilib>:"Write Delimited Spreadsheet.vi"("file path (dialog if empty)"=w589, "2D data"=w590) -> ()  [unwired: 12 in, 2 out]
            }
          }
        }
      }
      frame "save all" {
        n217 = property on="Z Slice" class="Slide (strict)"() -> ("Scale.Maximum"=w612:dbl)  [unwired: 2 in, 2 out]
        n218 = property on="ROIs List" class="Ring (strict)"() -> ("Strings []"=w600:string[])  [unwired: 2 in, 2 out]
        n219 = Array Size(array=w600) -> (size(s)=w609:i32)
        n220 = To Long Integer(number=w612) -> (32bit integer=w611:i32)
        n221 = Delete From Array(array=w600, index=0 ("index (row)")) -> (deleted portion=→"deleted portion 2":string, array with subset deleted=w599:string[])  [unwired: 1 in]
        n222 = Decrement(x=w611) -> (x-1=w610:i32)
        n223 = Decrement(x=w609) -> (x-1=w606:i32)
        n224 = Delete From Array(array=w605, index (row)=0) -> (deleted portion=→"deleted portion":i32[], array with subset deleted=w603:i32[][])  [unwired: 2 in]
        n225 = property on="Data Form" class="Clust (strict)"() -> ("Value"=w614:T2)  [unwired: 2 in, 2 out]
        n226 = for {
          N: w606 -> [_]
          tunnel: w616 -> [w626]
          tunnel: w614 -> [w625]
          tunnel: w603 -> [w624]
          tunnel: w610 -> [w622]
          shift-right: [w623] -> w613
          shift-left: w617 -> [w627]
          tunnel: w599 -> [w620] mode=indexing
          tunnel: w597 -> [w619]
          i -> [w621]
          n227 = case shown="False" w626 {
            selector: w626 -> [w632 w656]
            tunnel: w624 -> [w636 w660]
            tunnel: w627 -> [w630 w653]
            tunnel: w625 -> [w635 w655]
            tunnel: [w629 w652] -> w623
            tunnel: w622 -> [w634 _]
            tunnel: w621 -> [w633 w659]
            tunnel: w620 -> [w631 w654]
            tunnel: w619 -> [w628 w651]
            frame False {
              n228 = for {
                N: w634 -> [_]
                tunnel: w636 -> [w650]
                tunnel: w635 -> [w646]
                tunnel: w633 -> [w648]
                tunnel: w632 -> [w645]
                tunnel: w631 -> [w644]
                shift-right: [w642] -> w629
                shift-left: w630 -> [w643]
                tunnel: w628 -> [w638]
                i -> [w641]
                w637 = T4."Enabled" ("Disabled")
                n229 = call "extract roi 3d.vi"("ROI selected"=w648, "ROIs Array In"=w650, "Data Form"=w646) -> ("Table ROI 3D"=w649:i32[][][])  [unwired: 8 in]
                n230 = Index Array(array=w649, index (dim 0)=w641) -> (element=w647:i32[][])  [unwired: 2 in]
                n231 = Number To Decimal String(number=w641) -> (decimal integer string=w640:string)  [unwired: 1 in]
                n232 = call "name tables.vi"("2D?"=w645, "error in"=w643, "Z Slice"=w640, "ROI"=w644, "path folder in"=w638) -> ("error out"=w642:errorcluster, "path file out"=w639:path)  [unwired: 5 in]
                n233 = property on="Crop Z sl" class="Slide (strict)"("DisabledEnum"=w637) -> ()  [unwired: 2 in, 2 out]
                n234 = property on="crop Z" class="Bool"("DisabledEnum"=w637) -> ()  [unwired: 2 in, 2 out]
                n235 = call-poly <vilib>:"Write Delimited Spreadsheet.vi"("file path (dialog if empty)"=w639, "2D data"=w647) -> ()  [unwired: 12 in, 2 out]
              }
            }
            frame True {
              n236 = call "extract roi 2d.vi"("ROI selected"=w659, "ROIs Array In"=w660, "Data Form"=w655) -> ("Table ROI 2D"=w658:i32[][])  [unwired: 8 in]
              n237 = call "name tables.vi"("2D?"=w656, "error in"=w653, "ROI"=w654, "path folder in"=w651) -> ("error out"=w652:errorcluster, "path file out"=w657:path)  [unwired: 6 in]
              n238 = call-poly <vilib>:"Write Delimited Spreadsheet.vi"("file path (dialog if empty)"=w657, "2D data"=w658) -> ()  [unwired: 12 in, 2 out]
            }
          }
        }
      }
      frame "crop z" {
        n239 = Variant To Data(error in=w672, type=cluster{"sl1":i32, "sl2":i32} {"sl1"=0, "sl2"=3} ("Crop Z"), Variant=w671) -> (data=w661:cluster{"sl1":i32, "sl2":i32}, error out=w664:errorcluster)
        n240 = call "delete z slices tabs.vi"("error in"=w664, "Crop Z"=w661, "File Table Folder"=w662) -> ("error out"=w663:errorcluster)  [unwired: 8 in]
      }
      frame "zslice" {
        n241 = Variant To Data(error in=w683, type=cluster{"NewVal":i16, "ROIs List":i16} {"NewVal"=0, "ROIs List"=0} ("output cluster"), Variant=w682) -> (data=w679:cluster{"NewVal":i16, "ROIs List":i16}, error out=w681:errorcluster)
        n242 = Unbundle(w679) -> ("NewVal"=w678:i16, "ROIs List"=w677:i16)
        n243 = property on="Data Form" class="Clust (strict)"() -> ("Value"=w688:T2)  [unwired: 2 in, 2 out]
        n244 = call "extract roi 3d.vi"("ROI selected"=w677, "ROIs Array In"=w685, "Data Form"=w688) -> ("Table ROI 3D"=w684:i32[][][])  [unwired: 8 in]
        n245 = Index Array(array=w684, index (dim 0)=w678) -> (element=w689:i32[][])  [unwired: 2 in]
        n246 = property on="Intensity Graph" class="IntGraph (strict)"("Value"=w689) -> ()  [unwired: 2 in, 2 out]
      }
      frame "manipulate" {
        n247 = call "manipulate files.vi"("error in"=w696) -> ("error out"=w695:errorcluster)  [unwired: 10 in]
      }
      frame "export" {
        n248 = case shown="False" w701 {
          tunnel: w704 -> [w711 w714]
          tunnel: [w710 w713] -> w703
          tunnel: w700 -> [w709 w712]
          frame False {
            n249 = call "elab pictures 3d.vi"("error in"=w711, "path file in"=w709) -> ("error out"=w710:errorcluster)  [unwired: 9 in]
          }
          frame True {
            n250 = call "elab pictures 2d.vi"("error in"=w714, "path file in"=w712) -> ("error out"=w713:errorcluster)  [unwired: 9 in]
          }
        }
      }
    }
    "XY Graph" <- w16
  }
  "error out" <- w5
  n251 = while {
    tunnel: w3 -> [w720]
    tunnel: w7 -> [w719]
    shift-right: [w718] -> _
    shift-left: i16 0 ("ROIs List") -> [w717]
    shift-right: [w716] -> _
    shift-left: i16 0 ("NewVal") -> [w715]
    stop <- w721 stop-if-true
    n252 = event shown="[14] \"save\": Value Change" {
      selector: _ -> [_ _ _ _ _ _ _ _ _ _ _ _ _ _ _ _ _ _ _ _]
      dyn-events: _ -> [_ _ _ _ _ _ _ _ _ _ _ _ _ _ _ _ _ _ _ _]
      timeout: _ -> [_ _ _ _ _ _ _ _ _ _ _ _ _ _ _ _ _ _ _ _]
      tunnel: [FALSE TRUE FALSE FALSE FALSE FALSE FALSE FALSE FALSE FALSE FALSE FALSE FALSE FALSE FALSE FALSE FALSE FALSE FALSE FALSE] -> w721
      tunnel: w720 -> [_ w736 w744 w762 w771 _ w782 w789 w796 w805 w813 w828 w845 w856 w865 w872 w881 w888 w895 w901]
      tunnel: w719 -> [_ w730 w745 w760 w772 _ w783 w790 w797 w806 w814 w818 w846 w857 w866 w873 w882 w889 w896 w899]
      tunnel: [w723 w726 w738 w764 w767 w776 w778 w785 w792 w800 w808 w821 w848 w852 w861 w868 w877 w884 w891 w903] -> w718
      tunnel: w717 -> [w723 w726 w738 w764 w767 w776 w778 w785 w792 w800 _ w822 w848 w852 w861 w868 w877 w884 w891 w903]
      tunnel: [w722 w725 w737 w763 w766 w773 w777 w784 w791 w798 w809 w825 w849 w853 w862 w869 w878 w885 w892 w902] -> w716
      tunnel: w715 -> [w722 w725 w737 w763 w766 w773 w777 w784 w791 _ w809 w825 w849 w853 w862 w869 w878 w885 w892 w902]
      event Timeout {
        n253 = event-data() -> ()  [unwired: 1 in, 3 out]
      }
      event "Stop": Value Change {
        w727 = TRUE
        w733 = "stop" ("Message")
        n254 = event-data() -> ()  [unwired: 1 in, 4 out]
        n255 = Unbundle By Name(w736) -> ("Main"=w734:refnum<queue>, "2d"=w732:refnum<queue>, "3d"=w731:refnum<queue>)
        n256 = call "Enqueue Message (Single).vi"("Priority Message? (F)"=w727, "error in (no error)"=w730, "Message"=w733, "Message Queue"=w734) -> ("error out"=w729:errorcluster)  [unwired: 6 in, 1 out]
        n257 = call "Enqueue Message (Single).vi"("Priority Message? (F)"=w727, "error in (no error)"=w729, "Message"=w733, "Message Queue"=w732) -> ("error out"=w728:errorcluster)  [unwired: 6 in, 1 out]
        n258 = call "Enqueue Message (Single).vi"("Priority Message? (F)"=w727, "error in (no error)"=w728, "Message"=w733, "Message Queue"=w731) -> ()  [unwired: 6 in, 2 out]
      }
      event Value Change {
        w743 = "data form"
        n259 = event-data() -> ("NewVal"=w751:T2)  [unwired: 1 in, 3 out]
        n260 = Unbundle By Name("Data Form") -> ("Dimensions.Dim Z"=w740:i32)
        n261 = Less Or Equal To 0?(x=w740) -> (x <= 0?=w741:bool)
        n262 = case shown="False" w741 {
          tunnel: [w755 w758] -> w752
          tunnel: w744 -> [w756 w757]
          tunnel: w740 -> [w754 _]
          tunnel: T4."Enabled" ("Disabled") -> [w753 _]
          frame False {
            n263 = property on="Z Slice" class="Slide (strict)"("DisabledEnum"=w753, "Scale.Maximum"=w754) -> ()  [unwired: 2 in, 2 out]
            n264 = Unbundle By Name(w756) -> ("3d"=w755:refnum<queue>)
          }
          frame True {
            n265 = Unbundle By Name(w757) -> ("2d"=w758:refnum<queue>)
          }
        }
        n266 = To Variant(anything=w751) -> (Variant=w750:variant)
        n267 = Unbundle By Name(w744) -> ("Main"=w747:refnum<queue>)
        n268 = call "Enqueue Message (Single).vi"("error in (no error)"=w745, "Message Data"=w750, "Message"=w743, "Message Queue"=w752) -> ("error out"=w742:errorcluster)  [unwired: 6 in, 1 out]
        n269 = To Variant(anything=w741) -> (Variant=w746:variant)
        n270 = call "Enqueue Message (Single).vi"("error in (no error)"=w742, "Message Data"=w746, "Message"=w743, "Message Queue"=w747) -> ()  [unwired: 6 in, 2 out]
      }
      event Value Change {
        n271 = event-data() -> ()  [unwired: 1 in, 4 out]
        n272 = Unbundle By Name(w762) -> ("Main"=w761:refnum<queue>)
        n273 = call "Enqueue Message (Single).vi"("error in (no error)"=w760, "Message"="folder tabs", "Message Queue"=w761) -> ()  [unwired: 7 in, 2 out]
      }
      event "load data": Value Change {
        n274 = event-data() -> ()  [unwired: 1 in, 6 out]
        n275 = Unbundle By Name(w771) -> ("Main"=w770:refnum<queue>)
        n276 = call "Enqueue Message (Single).vi"("error in (no error)"=w772, "Message"="load data", "Message Queue"=w770) -> ()  [unwired: 7 in, 2 out]
      }
      event "mapping": Value Change {
        n277 = event-data() -> ("NewVal"=w774:enum16{"Y - Linear", "Y - Log"})  [unwired: 1 in, 5 out]
        n278 = property on="XY Graph" class="XYGraph (strict)"("YScale.Mapping Mode"=w774) -> ()  [unwired: 2 in, 2 out]
      }
      event "calibrate": Value Change {
        n279 = event-data() -> ()  [unwired: 1 in, 6 out]
        n280 = Unbundle By Name(w782) -> ("Main"=w781:refnum<queue>)
        n281 = call "Enqueue Message (Single).vi"("error in (no error)"=w783, "Message"="calibrate", "Message Queue"=w781) -> ()  [unwired: 7 in, 2 out]
      }
      event "load calib": Value Change {
        n282 = event-data() -> ()  [unwired: 1 in, 6 out]
        n283 = Unbundle By Name(w789) -> ("Main"=w788:refnum<queue>)
        n284 = call "Enqueue Message (Single).vi"("error in (no error)"=w790, "Message"="load calib", "Message Queue"=w788) -> ()  [unwired: 7 in, 2 out]
      }
      event "load param": Value Change {
        n285 = event-data() -> ()  [unwired: 1 in, 6 out]
        n286 = Unbundle By Name(w796) -> ("Main"=w795:refnum<queue>)
        n287 = call "Enqueue Message (Single).vi"("error in (no error)"=w797, "Message"="load parameters", "Message Queue"=w795) -> ()  [unwired: 7 in, 2 out]
      }
      event "Z Slice": Value Change {
        n288 = event-data() -> ("NewVal"=w798:i16)  [unwired: 1 in, 3 out]
        n289 = Bundle("NewVal"=w798, "ROIs List"=w800) -> (w799:cluster{"NewVal":i16, "ROIs List":i16})  [unwired: 1 in]
        n290 = To Variant(anything=w799) -> (Variant=w802:variant)
        n291 = Unbundle By Name(w805) -> ("Main"=w804:refnum<queue>)
        n292 = call "Enqueue Message (Single).vi"("error in (no error)"=w806, "Message Data"=w802, "Message"="zslice", "Message Queue"=w804) -> ()  [unwired: 6 in, 2 out]
      }
      event "ROIs List": Value Change {
        n293 = event-data() -> ("NewVal"=w808:i16)  [unwired: 1 in, 4 out]
        n294 = Unbundle By Name(w813) -> ("Main"=w812:refnum<queue>)
        n295 = Bundle("NewVal"=w809, "NewVal"=w808) -> (w807:cluster{"NewVal":i16, "NewVal":i16})  [unwired: 1 in]
        n296 = To Variant(anything=w807) -> (Variant=w811:variant)
        n297 = call "Enqueue Message (Single).vi"("error in (no error)"=w814, "Message Data"=w811, "Message"="roi", "Message Queue"=w812) -> ()  [unwired: 6 in, 2 out]
      }
      event "roi": Value Change {
        n298 = event-data() -> ()  [unwired: 1 in, 6 out]
        n299 = Unbundle By Name(w828) -> ("Main"=w817:refnum<queue>)
        n300 = Equal?(x=w822, y=i16 0) -> (x = y?=w816:bool)
        n301 = case shown="True" w816 {
          tunnel: w817 -> [w832 w837]
          tunnel: [w832 w837] -> w820
          tunnel: w818 -> [w831 w838]
          tunnel: [w831 w838] -> w819
          tunnel: w822 -> [w830 _]
          tunnel: [w830 w833] -> w821
          frame False {
          }
          frame True {
            n302 = property on="ROIs List" class="Ring (strict)"() -> ("NumItems"=w835:u32, "Strings []"=w840:string[])  [unwired: 2 in, 2 out]
            n303 = Number To Decimal String(number=w835) -> (decimal integer string=w841:string)  [unwired: 1 in]
            n304 = Concatenate Strings("ROI ", w841) -> (w836:string)
            n305 = Increment(x=w835) -> (x+1=w834:u32)
            n306 = Build Array (concatenate)(w840, w836) -> (w839:string[])
            n307 = To Word Integer(number=w834) -> (16bit integer=w833:i16)
            n308 = property on="ROIs List" class="Ring (strict)"("Strings []"=w839) -> ()  [unwired: 2 in, 2 out]
          }
        }
        n309 = Bundle("NewVal"=w825, "ROIs List"=w821, w816) -> (w824:cluster{"NewVal":i16, "ROIs List":i16, bool})  [unwired: 1 in]
        n310 = To Variant(anything=w824) -> (Variant=w827:variant)
        n311 = call "Enqueue Message (Single).vi"("error in (no error)"=w819, "Message Data"=w827, "Message"="edit roi", "Message Queue"=w820) -> ()  [unwired: 6 in, 2 out]
      }
      event "manipulate files": Value Change {
        n312 = event-data() -> ()  [unwired: 1 in, 5 out]
        n313 = Unbundle By Name(w845) -> ("Main"=w844:refnum<queue>)
        n314 = call "Enqueue Message (Single).vi"("error in (no error)"=w846, "Message"="manipulate", "Message Queue"=w844) -> ()  [unwired: 7 in, 2 out]
      }
      event "crop": Value Change {
        n315 = event-data() -> ()  [unwired: 1 in, 5 out]
        n316 = Bundle("NewVal"=w853, "ROIs List"=w852) -> (w851:cluster{"NewVal":i16, "ROIs List":i16})  [unwired: 1 in]
        n317 = To Variant(anything=w851) -> (Variant=w850:variant)
        n318 = Unbundle By Name(w856) -> ("Main"=w855:refnum<queue>)
        n319 = call "Enqueue Message (Single).vi"("error in (no error)"=w857, "Message Data"=w850, "Message"="crop", "Message Queue"=w855) -> ()  [unwired: 6 in, 2 out]
      }
      event "save": Value Change {
        n320 = event-data() -> ()  [unwired: 1 in, 5 out]
        n321 = Bundle("NewVal"=w862, "ROIs List"=w861) -> (w860:cluster{"NewVal":i16, "ROIs List":i16})  [unwired: 1 in]
        n322 = To Variant(anything=w860) -> (Variant=w859:variant)
        n323 = Unbundle By Name(w865) -> ("Main"=w864:refnum<queue>)
        n324 = call "Enqueue Message (Single).vi"("error in (no error)"=w866, "Message Data"=w859, "Message"="save", "Message Queue"=w864) -> ()  [unwired: 6 in, 2 out]
      }
      event "crop all": Value Change {
        n325 = event-data() -> ()  [unwired: 1 in, 5 out]
        n326 = Unbundle By Name(w872) -> ("Main"=w871:refnum<queue>)
        n327 = call "Enqueue Message (Single).vi"("error in (no error)"=w873, "Message"="crop all", "Message Queue"=w871) -> ()  [unwired: 7 in, 2 out]
      }
      event "crop Z": Value Change {
        n328 = event-data() -> ()  [unwired: 1 in, 5 out]
        n329 = To Variant(anything="Crop Z sl") -> (Variant=w875:variant)
        n330 = Unbundle By Name(w881) -> ("Main"=w880:refnum<queue>)
        n331 = call "Enqueue Message (Single).vi"("error in (no error)"=w882, "Message Data"=w875, "Message"="crop z", "Message Queue"=w880) -> ()  [unwired: 6 in, 2 out]
      }
      event "save all": Value Change {
        n332 = event-data() -> ()  [unwired: 1 in, 5 out]
        n333 = Unbundle By Name(w888) -> ("Main"=w887:refnum<queue>)
        n334 = call "Enqueue Message (Single).vi"("error in (no error)"=w889, "Message"="save all", "Message Queue"=w887) -> ()  [unwired: 7 in, 2 out]
      }
      event "reset ROI": Value Change {
        n335 = event-data() -> ()  [unwired: 1 in, 5 out]
        n336 = Unbundle By Name(w895) -> ("Main"=w894:refnum<queue>)
        n337 = call "Enqueue Message (Single).vi"("error in (no error)"=w896, "Message"="reset roi", "Message Queue"=w894) -> ()  [unwired: 7 in, 2 out]
      }
      event "export": Value Change {
        n338 = event-data() -> ()  [unwired: 1 in, 3 out]
        n339 = Unbundle By Name(w901) -> ("Main"=w900:refnum<queue>)
        n340 = call "Enqueue Message (Single).vi"("error in (no error)"=w899, "Message"="export", "Message Queue"=w900) -> ()  [unwired: 7 in, 2 out]
      }
    }
  }
